vi "Setup.vi"(11 "TEMPLATE jettl in":refnum<class "TEMPLATE jettl.lvclass">) -> (3 "TEMPLATE jettl out":refnum<class "TEMPLATE jettl.lvclass">)   [LabVIEW 2021, in "_Template.lvlib" / "Templates.lvlib" / "TEMPLATE jettl.lvlib" / "TEMPLATE jettl.lvclass"]
uses:
  TEMPLATE jettl.lvclass
  TEMPLATE jettl.lvclass/TEMPLATE jettl.ctl
  jettl/jettl/jettl/jettl.lvclass
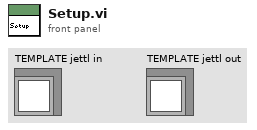
[diagram p1: front panel]
types:
  T1 = enum32{"Invalid", "Standard", "Closed", "Hidden", "Minimized", "Maximized"}
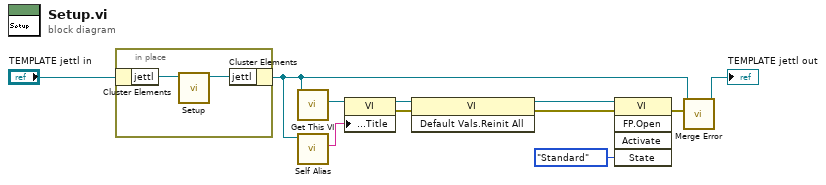
[diagram p0: block diagram]
diagram:
  n1 = in-place {
    n2 = in-place-cluster #1("TEMPLATE jettl in") -> ("jettl"=w13:refnum<class "jettl.lvclass">)
    n3 = call-dynamic "Setup.vi"("Setup in"=w13) -> ("Setup out"=w12:refnum<class "jettl.lvclass">)  [unwired: 10 in]
    n4 = in-place-cluster #1("jettl"=w12) -> (w4:refnum<class "TEMPLATE jettl.lvclass">)
  }
  n5 = call-dynamic "Get This VI.vi"("TEMPLATE jettl in"=w4) -> ("This VI"=w3:refnum<vi>)  [unwired: 10 in]
  n6 = call-dynamic "Self Alias.vi"("TEMPLATE jettl in"=w4) -> ("Self Alias"=w5:string)  [unwired: 9 in, 1 out]
  n7 = property class="VI"(reference=w3, "Front Panel.Title"=w5) -> (reference out=w2:refnum<vi>, error out=w1:errorcluster)  [unwired: 1 in]
  n8 = invoke class="VI" method="Default Vals.Reinit All"(reference=w2, error in=w1) -> (reference out=w6:refnum<vi>, error out=w7:errorcluster)  [unwired: 1 in, 1 out]
  n9 = invoke class="VI" method="FP.Open"(reference=w6, error in=w7, "State"=T1."Standard") -> (error out=w8:errorcluster)  [unwired: 2 in, 4 out]
  n10 = call-dynamic "Merge Error.vi"("Error"=w8, "TEMPLATE jettl in"=w4) -> ("TEMPLATE jettl out"=→"TEMPLATE jettl out":refnum<class "TEMPLATE jettl.lvclass">)  [unwired: 9 in]
